vi "_CSMObj-Enqueue Cross-Module Message.vi"(8 "Error In":errorcluster caption="error in (no error)", 9 "High Priority? (F)":bool, 10 "Data":T1, 11 "CSMQ In":T4={"info"={"Module Name"="", "Requested Name"="", "Group Name"="", "Mode"=enum."Stand Alone", "Allowed Messages"=[]}, "Refs"={"WatchDogQ"=refnum, "CSMDataDVR"=refnum, "Queue"={"HPriorityQ"=refnum, "LowPriorityQ"=refnum}, "GroupDataDVR"=refnum, "TagMap"=refnum, "ExitEvent"=refnum, "NewStateEvent"=refnum, "StatusEvent"=refnum, "InterruptEvent"=refnum}}) -> (0 "error out":errorcluster, 3 "CSMQ Out":T4={"info"={"Module Name"="", "Requested Name"="", "Group Name"="", "Mode"=enum."Stand Alone", "Allowed Messages"=[]}, "Refs"={"WatchDogQ"=refnum, "CSMDataDVR"=refnum, "Queue"={"HPriorityQ"=refnum, "LowPriorityQ"=refnum}, "GroupDataDVR"=refnum, "TagMap"=refnum, "ExitEvent"=refnum, "NewStateEvent"=refnum, "StatusEvent"=refnum, "InterruptEvent"=refnum}})   [LabVIEW 2017, in "Communicable State Machine.lvlib"]
uses:
  Communicable State Machine.lvlib
  _CSMObj.ctl
  _CSMObj-Info.ctl
  Typedef/_CSM_MODE.ctl
  _CSMObj-Refs.ctl
  _CSMObj-Data.ctl
  Priority Queue/Priority Queue.ctl
  Typedef/_Cross CSM State Data.ctl
  Typedef/_CSM_MSG_TYPE.ctl
  Typedef/_Cross CSM State Response.ctl
  Typedef/_CSM_Response Source Message.ctl
  Priority Queue/def-Data(LowPRI-Q).ctl
  _CSMObj-ModeData.ctl
  Typedef/_CSM Status Change Event Data.ctl
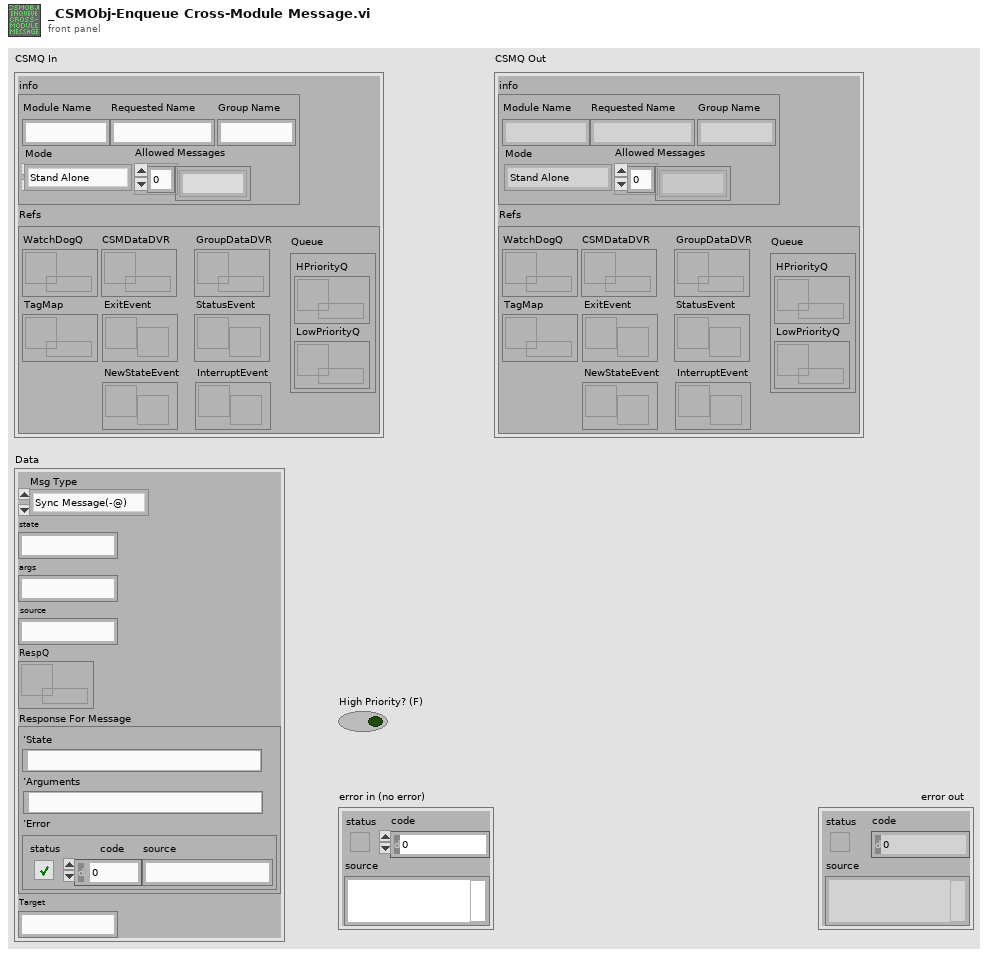
[diagram p1: front panel]
types:
  T1 = typedef "Communicable State Machine.lvlib/_Cross CSM State Data.ctl" = cluster{"Msg Type":T2, "state":string, "args":string, "source":string, "RespQ":refnum<queue>, "Response For Message":T3, "Target":string}
  T2 = typedef "Communicable State Machine.lvlib/_CSM_MSG_TYPE.ctl" = enum16{"Sync Message(-@)", "Async Message(->)", "Async without Response(->|)", "Async Response", "Broadcast(-><all>)", "Broadcast(-><status>)", "Broadcast(-><interrupt>)", "Append to JKISM States", "Append to JKISM States(High Priority)", "Broadcast(-><state>)"}
  T3 = typedef "Communicable State Machine.lvlib/_CSM_Response Source Message.ctl" = cluster{"‘State":string, "’Arguments":string, "’Error":errorcluster}
  T4 = typedef "Communicable State Machine.lvlib/_CSMObj.ctl" = cluster{"info":T5, "Refs":T7}
  T5 = typedef "Communicable State Machine.lvlib/_CSMObj-Info.ctl" = cluster{"Module Name":string, "Requested Name":string, "Group Name":string, "Mode":T6, "Allowed Messages":string[]}
  T6 = typedef "Communicable State Machine.lvlib/_CSM_MODE.ctl" = enum16{"Not Exist", "Stand Alone", "CSM", "Worker", "Worker Agent", "Chain Node", "Chain"}
  T7 = typedef "Communicable State Machine.lvlib/_CSMObj-Refs.ctl" = cluster{"WatchDogQ":refnum<queue>, "CSMDataDVR":refnum<data-value>, "Queue":T8, "GroupDataDVR":refnum<data-value>, "TagMap":refnum<data-value>, "ExitEvent":refnum<user-event>, "NewStateEvent":refnum<user-event>, "StatusEvent":refnum<user-event>, "InterruptEvent":refnum<user-event>}
  T8 = typedef "Communicable State Machine.lvlib/Priority Queue.ctl" = cluster{"HPriorityQ":refnum<queue>, "LowPriorityQ":refnum<queue>}
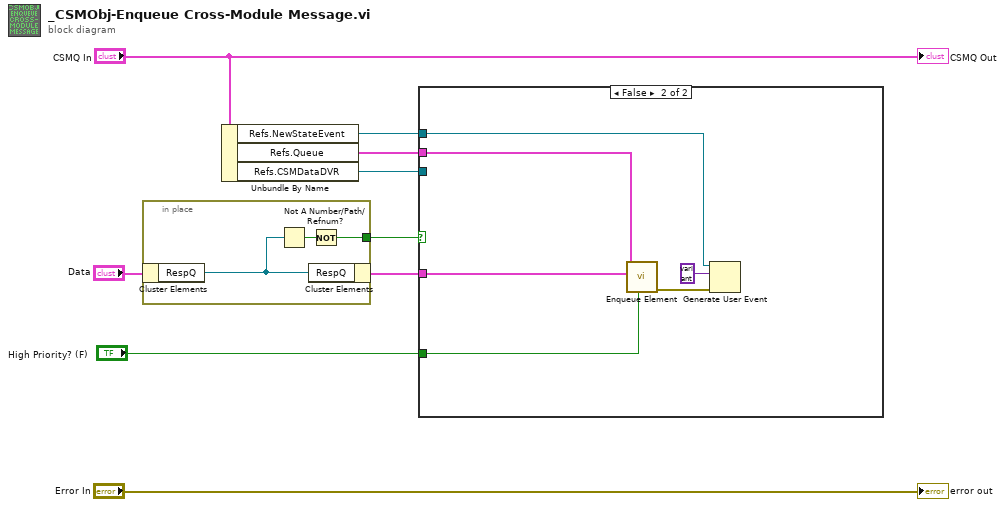
[diagram p0: block diagram]
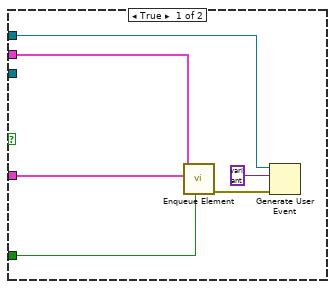
[diagram p2: hidden frame]
diagram:
  n1 = in-place {
    in-place-border: [w10] -> w5
    n2 = in-place-cluster #1("Data") -> ("RespQ"=w12:refnum<queue>)
    n3 = Not A Number/Path/Refnum?(number/path/refnum=w12) -> (NaN/Path/Refnum?=w11:bool)
    n4 = in-place-cluster #1("RespQ"=w12) -> (w6:T1)
    n5 = Not(x=w11) -> (.not. x?=w10:bool)
  }
  n6 = Unbundle By Name("CSMQ In") -> ("Refs.NewStateEvent"=w2:refnum<user-event>, "Refs.Queue"=w7:T8, "Refs.CSMDataDVR"=w4:refnum<data-value>)
  n7 = case shown="False" w5 {
    tunnel: w7 -> [w18 w24]
    tunnel: w6 -> [w17 w23]
    tunnel: w4 -> [_ _]
    tunnel: w2 -> [w16 w20]
    tunnel: "High Priority? (F)" -> [w15 w19]
    frame True {
      n8 = call "Enqueue Element.vi"("High Priority? (F)"=w15, "Cross JKI State Machine State"=w17, "Priority Queue"=w18) -> ("error out"=w14:errorcluster)  [unwired: 7 in, 1 out]
      n9 = Generate User Event(user event=w16, event data cluster=variant ("event data"), error in=w14) -> ()  [unwired: 1 in, 2 out]
    }
    frame False {
      n10 = call "Enqueue Element.vi"("High Priority? (F)"=w19, "Cross JKI State Machine State"=w23, "Priority Queue"=w24) -> ("error out"=w21:errorcluster)  [unwired: 7 in, 1 out]
      n11 = Generate User Event(user event=w20, event data cluster=variant ("event data"), error in=w21) -> ()  [unwired: 1 in, 2 out]
    }
  }
  "error out" <- "Error In"
  "CSMQ Out" <- "CSMQ In"
